vi "Test Count Errors on Broken.vi"(8 "error in (no error)":errorcluster, 11 "Result Model Tests in":refnum<class "Result Model Test Enumeration.lvclass">) -> (0 "error out":errorcluster, 3 "Result Model Tests out":refnum<class "Result Model Test Enumeration.lvclass">)   [LabVIEW 2020, in "Result Model Test Enumeration.lvclass"]
uses:
  Result Model Test Enumeration.lvclass
  Result Model Test Enumeration.lvclass/Result Model Test Enumeration.ctl
  206db1ee-aa99-40b9-8881-171f2a77c34b.vi
  Result Model/Result Model.lvclass
  Result/Type.ctl
  Result/Result.lvlib
  Result/Status.ctl
  Result/Result.ctl
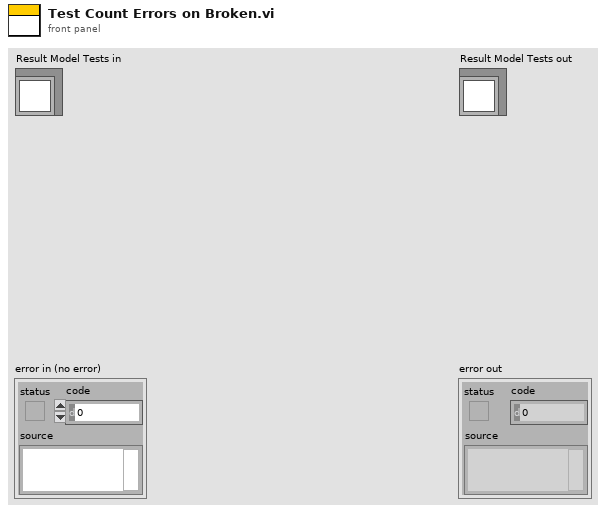
[diagram p1: front panel]
types:
  T1 = typedef "Result.lvlib/Result.ctl" = cluster{"Name":string, "Message":string, "Description":string, "Status":T2, "Result Type":T3, "Execution Time":dbl}
  T2 = typedef "Result.lvlib/Status.ctl" = enum16{"", "Passed", "Failed", "Error", "Skipped", "Setup Error", "Broken", "Teardown Error"}
  T3 = typedef "Result.lvlib/Type.ctl" = enum16{"Method", "Case", "Suite", "Pass", "Fail", "Skip", "Pass if", "Fail if", "Pass if Error", "Fail if Error", "Pass if Equal", "Fail if Equal"}
  T4 = typedef "Result Model.lvclass/Statistics.ctl" = cluster{"Method Count":u32, "Executed Methods":u32, "Passed Methods":u32, "Failed Methods":u32, "Method Errors":u32, "Skipped Method":u32}
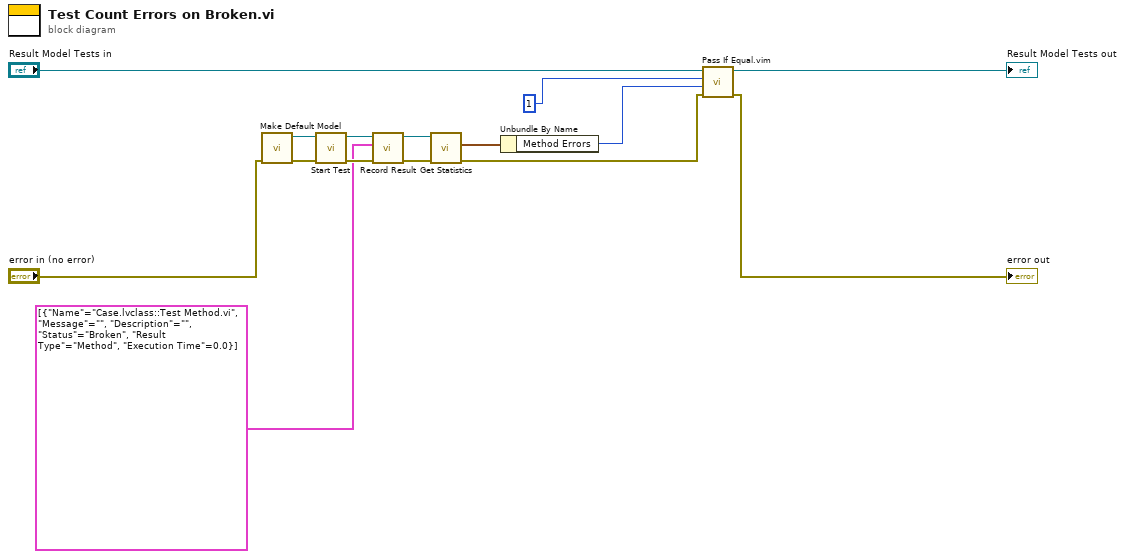
[diagram p0: block diagram]
diagram:
  n1 = call "Make Default Model.vi"("error in (no error)"="error in (no error)") -> ("error out"=w13:errorcluster, "Result Model out"=w14:refnum<class "Result Model.lvclass">)  [unwired: 9 in]
  n2 = call "Start Test.vi"("error in (no error)"=w13, "Result Model In"=w14) -> ("error out"=w8:errorcluster, "Result Model Out"=w3:refnum<class "Result Model.lvclass">)  [unwired: 8 in]
  n3 = call "Record Result.vi"("error in (no error)"=w8, "Results"=T1[] [{"Name"="Case.lvclass::Test Method.vi", "Message"="", "Description"="", "Status"=enum."Broken", "Result Type"=enum."Method", "Execution Time"=0.0}], "Result Model in"=w3) -> ("error out"=w4:errorcluster, "Result Model out"=w2:refnum<class "Result Model.lvclass">)  [unwired: 7 in]
  n4 = call "Get Statistics.vi"("error in (no error)"=w4, "Result Model in"=w2) -> ("error out"=w10:errorcluster, "Results"=w7:T4)  [unwired: 7 in, 1 out]
  n5 = Unbundle By Name(w7) -> ("Method Errors"=w6:u32)
  n6 = call "Pass If Equal.vim"("error in (no error)"=w10, "Actual"=w6, "Expected"=u32 1 ("Method Count"), "LUnit Test Case In"="Result Model Tests in") -> ("error out"=→"error out":errorcluster, "LUnit Test Case Out"=→"Result Model Tests out":refnum<class "Result Model Test Enumeration.lvclass">)  [unwired: 6 in]
